vi "includePhysicalChannelsIntoData.vi"(8 "error in (no error)":errorcluster, 11 "SoundAO in":refnum<class "SoundAO.lvclass">) -> (0 "error out":errorcluster, 2 "transformedData":dbl[][](array[numeric]), 3 "SoundAO out":refnum<class "SoundAO.lvclass">)   [LabVIEW 2011, in "Hardware.lvlib" / "Channels.lvlib" / "SoundAO.lvclass"]
uses:
  SoundAO.lvclass
  AnalogOutput.lvclass
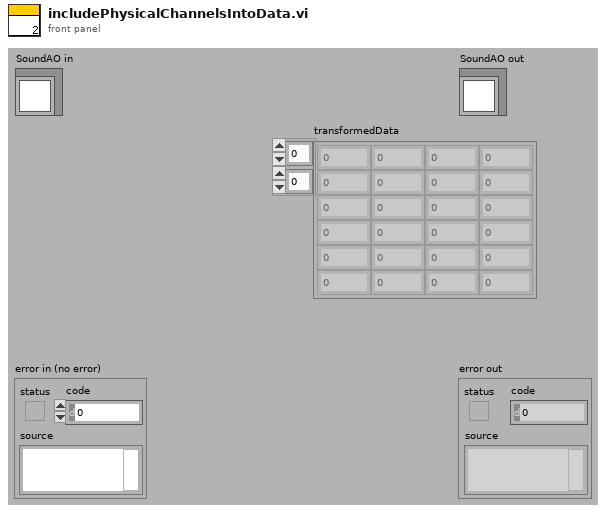
[diagram p1: front panel]
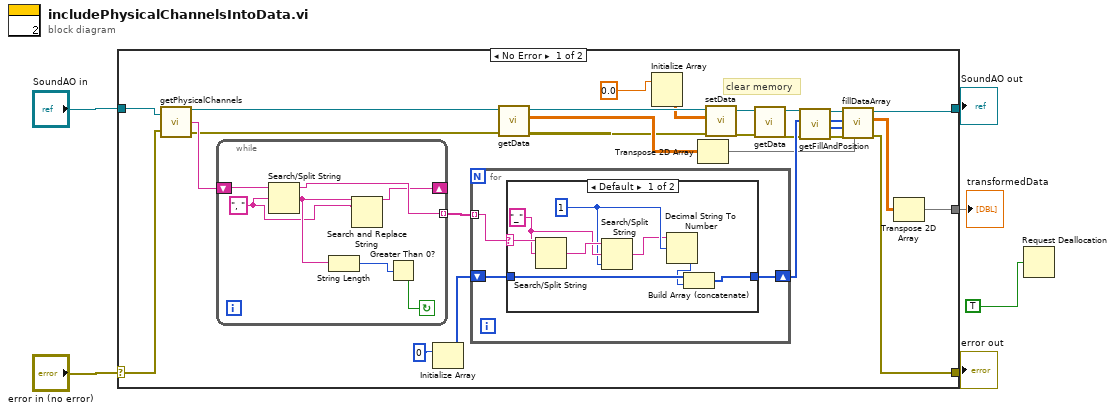
[diagram p0: block diagram]
diagram:
  n1 = case shown="No Error" "error in (no error)" {
    selector: "error in (no error)" -> [w29 w54]
    tunnel: [w21 w54] -> w5
    tunnel: [w22 w53] -> w3
    tunnel: "SoundAO in" -> [w30 w53]
    tunnel: [w15 _] -> w2
    frame No Error {
      # "clear memory"
      n2 = call-dynamic "getPhysicalChannels.vi"("AnalogOutput.lvclass in"=w30, "error in (no error)"=w29) -> ("AnalogOutput.lvclass out"=w20:refnum<class "SoundAO.lvclass">, "Physical Channels"=w28:string, "error out"=w19:errorcluster)
      n3 = while {
        shift-right: [w48] -> _
        shift-left: w28 -> [w52]
        tunnel: [w51] -> w33 mode=indexing
        stop <- w46 continue-if-true
        w49 = ", "
        n4 = Search/Split String(string=w52, search string/char (-)=w49) -> (substring before match=w51:string, match + rest of string=w50:string)  [unwired: 1 in, 1 out]
        n5 = String Length(string=w50) -> (length=w47:i32)
        n6 = Search and Replace String(input string=w50, search string=w49) -> (result string=w48:string)  [unwired: 6 in, 3 out]
        n7 = Greater Than 0?(x=w47) -> (x > 0?=w46:bool)
      }
      n8 = Initialize Array(0) -> (w32:i32[])  [unwired: 1 in]
      n9 = for {
        tunnel: w33 -> [w36] mode=indexing
        shift-right: [w34] -> w27
        shift-left: w32 -> [w35]
        n10 = case shown="Default" w36 {
          selector: w36 -> [w41 _]
          tunnel: w35 -> [w44 w45]
          tunnel: [w42 w45] -> w34
          frame Default {
            w38 = 1
            w39 = "_"
            n11 = Search/Split String(string=w41, search string/char (-)=w39) -> (match + rest of string=w40:string)  [unwired: 1 in, 2 out]
            n12 = Search/Split String(string=w40, search string/char (-)=w39, offset (0)=w38) -> (match + rest of string=w37:string)  [unwired: 2 out]
            n13 = Decimal String To Number(string=w37, offset=w38) -> (number=w43:i32)  [unwired: 1 in, 1 out]
            n14 = Build Array (concatenate)(w44, w43) -> (w42:i32[])
          }
          frame "" {
          }
        }
      }
      n15 = call "getData.vi"("error in (no error)"=w19, "AnalogOutput.lvclass in"=w20) -> ("error out"=w14:errorcluster, "Data"=w18:dbl[][], "AnalogOutput.lvclass out"=w13:refnum<class "SoundAO.lvclass">)  [unwired: 7 in]
      n16 = Initialize Array(0.0) -> (w11:dbl[][])  [unwired: 2 in]
      n17 = Transpose 2D Array(2D array=w18) -> (transposed array=w16:dbl[][])
      n18 = call "setData.vi"("error in (no error)"=w14, "Data"=w11, "AnalogOutput.lvclass in"=w13) -> ("error out"=w9:errorcluster, "AnalogOutput.lvclass out"=w10:refnum<class "SoundAO.lvclass">)  [unwired: 7 in]
      n19 = call "getData.vi"("error in (no error)"=w9, "AnalogOutput.lvclass in"=w10) -> ("error out"=w7:errorcluster, "AnalogOutput.lvclass out"=w8:refnum<class "SoundAO.lvclass">)  [unwired: 7 in, 1 out]
      n20 = call "getFillAndPosition.vi"("error in (no error)"=w7, "Array"=w27, "SoundAO in"=w8) -> ("error out"=w23:errorcluster, "fill number"=w24:i32[], "position"=w25:i32[], "SoundAO out"=w26:refnum<class "SoundAO.lvclass">)  [unwired: 5 in]
      n21 = call "fillDataArray.vi"("Data"=w16, "error in (no error)"=w23, "fill number"=w24, "position"=w25, "SoundAO in"=w26) -> ("error out"=w21:errorcluster, "transformedData"=w17:dbl[][], "SoundAO out"=w22:refnum<class "SoundAO.lvclass">)  [unwired: 4 in]
      n22 = Transpose 2D Array(2D array=w17) -> (transposed array=w15:dbl[][])
    }
    frame Error {
    }
  }
  "error out" <- w5
  "SoundAO out" <- w3
  "transformedData" <- w2
  n23 = Request Deallocation(TRUE) -> ()
